vi "AE Save-Kamronn-Medtech.vi"(0 "error in (no error)":errorcluster, 2 "LstBox Refnum":refnum<vi>, 3 "Variant In":variant, 4 "Action":T1=enum."Save Listbox") -> (7 "error out":errorcluster, 10 "Anything":variant)   [LabVIEW 2013, in "main.lvlib"]
uses:
  main.lvlib
  Controls/Enum Save Action Events.ctl
  Controls/SaveDataCluster.ctl
  Controls/Enum Variables.ctl
  <userlib>/_OpenG.lib/file/file.llb/Valid Path - Traditional__ogtk.vi
  <userlib>/_OpenG.lib/file/file.llb/File Exists - Scalar__ogtk.vi
  Globals/DataPathGlobalVariable.vi
  Globals/DataAcqRecordPathGlobal.vi
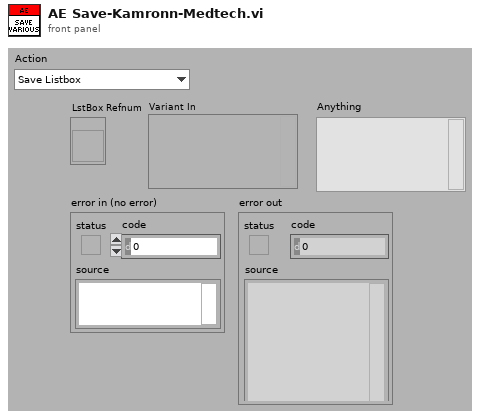
[diagram p1: front panel]
types:
  T1 = typedef "main.lvlib/Enum Save Action Events.ctl" = enum16{"LoadReportPath", "SaveReportPath", "Load Graph Path", "Save Graph Path", "LoadDataPath", "SaveDataPath", "Load Template Path", "Save Template Path", "Load PressureFactor", "Save PressureFactor", "Init", "Load Listbox", "Save Listbox", "LoadHospInfo", "SaveHospInfo", "Load DICOM Activation", "Save DICOM Activation", "LoadDICOMInfoWL", "SaveDICOMInfoWL", "LoadDICOMInfoPACS", "SaveDICOMInfoPACS", "Load ArmCalcMethod", "Save ArmCalcMethod", "LoadItemTags", "SaveItemTags", "LoadDICOMEncoding", "SaveDICOMEncoding", "LoadJournalType", "SaveJournalType", "LoadAcqFilterType", "SaveAcqFilterType", "Load Sequence", "Save Sequence", "Load Acquisition Mode", "Save Acquisition Mode", "Load General Settings", "Save General Settings", "Load Language", "Save Language", "Load Dicom Tags", "Save Dicom Tags", "Load BT Serial", "Save BT Serial", "Load BT License", "Save BT License"}
  T2 = typedef "main.lvlib/SaveDataCluster.ctl" = cluster{"HospInfo":cluster{"Name":string, "Address":string, "Department":string}, "Pressure":cluster{"Pressure":dbl}, "DataPath":cluster{"DataPath":path}, "ReportPath":cluster{"Path":path, "Name":string}, "DICOM Info WL":cluster{"port":i32, "AEtitle":string, "host":string, "remoteAE":string}, "DICOM Info PACS":cluster{"port":i32, "AEtitle":string, "host":string, "remoteAE":string}, "ArmCalcMethod":dbl, "itemTags":string[], "DicomEncoding":u16, "JournalType":u16, "General Settings":cluster{"Hyphenation":bool, "Language":u16, "CellStr1":string, "CellStr2":string}, "Dicom Tags":string[][], "BT Serial":cluster{"Serial Number":string, "Side":string, "Ignore?":bool}[], "BT License":cluster{"License":string, "Accepted Serials":string[]}}
  T3 = typedef "main.lvlib/Enum Variables.ctl" = enum16{"SetAcqFilter", "GetAcqFilter", "Set Filter", "Get Filter", "Set Height", "Get Height", "Set Recorded Height", "Get Recorded Height", "Set Blue Pressure", "Get Blue Pressure", "Set Red Pressure", "Get Red Pressure", "Init", "Reset Pressure", "Set Red Cursors", "Get Red Cursors", "Set Blue Cursors", "Get Blue Cursors", "Set Language", "Get Language", "Set Active Graphs", "Get ActiveGraphs", "Set Method", "Get Method", "Set Encryption", "Get Encryption", "Set ExcelVersion", "Get ExcelVersion", "Set DICOM Avail", "Get DICOM Avail", "Set DICOM Encode", "Get DICOM Encode", "Set JournalExport", "Get JournalExport", "Set Sequence", "Get Sequence", "Set DAQ Connected", "Get DAQ Connected", "Set Current Graph", "Get Current Graph", "Set General Settings", "Get Hyphenation", "Set Arm Calc Method", "Get Arm Calc Method", "Set Dicom Tags", "Get Dicom Tags", "Set BT Serial", "Get BT Serial", "Set BT Accepted Serials", "Get BT Accepted Serials", "Get BT License", "Set BT License"}
  T4 = cluster{"Name":string, "Address":string, "Department":string}
  T5 = cluster{"port":i32, "AEtitle":string, "host":string, "remoteAE":string}
  T6 = cluster{"Hyphenation":bool, "Language":u16, "CellStr1":string, "CellStr2":string}
  T7 = cluster{"Serial Number":string, "Side":string, "Ignore?":bool}[]
  T8 = cluster{"License":string, "Accepted Serials":string[]}
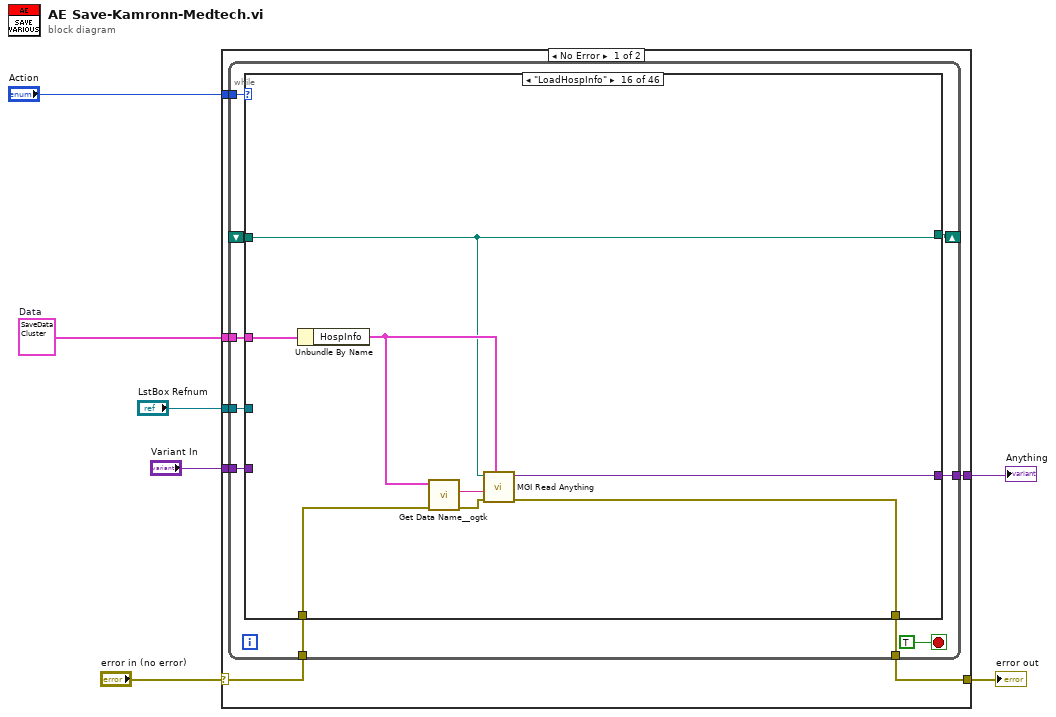
[diagram p0: block diagram]
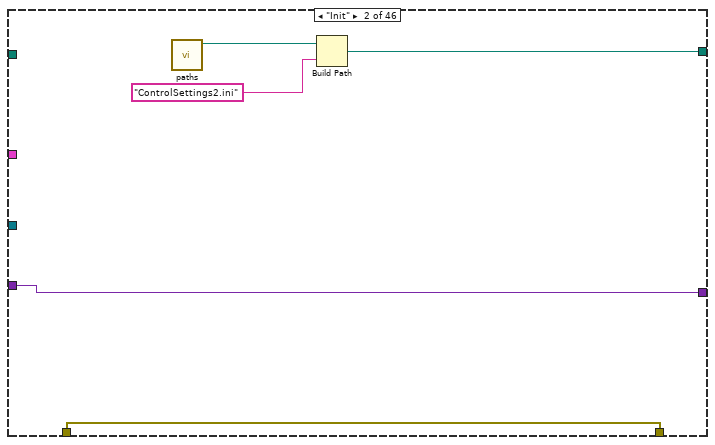
[diagram p3: hidden frame]
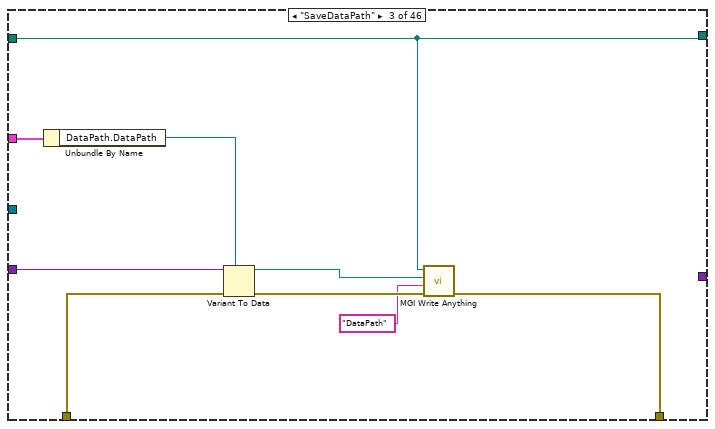
[diagram p4: hidden frame]
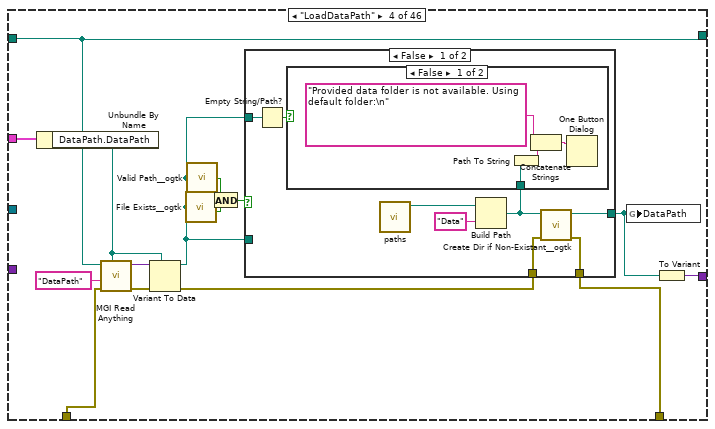
[diagram p5: hidden frame]
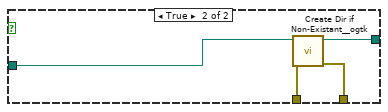
[diagram p7: hidden frame]
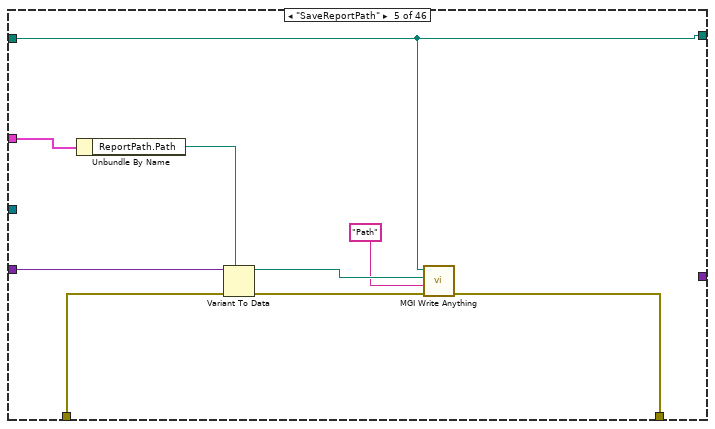
[diagram p8: hidden frame]
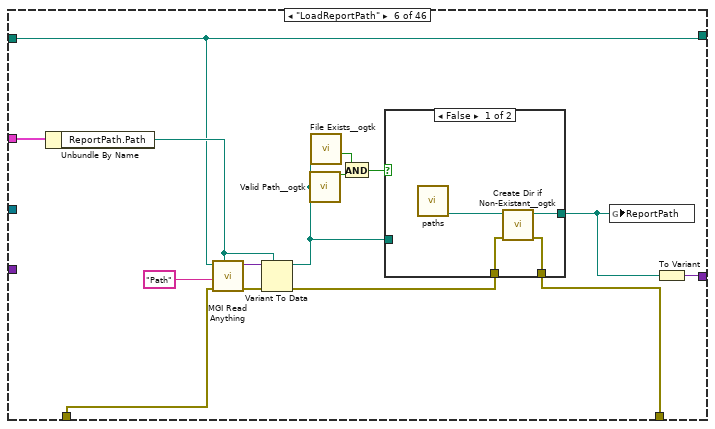
[diagram p9: hidden frame]
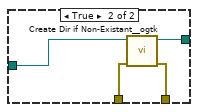
[diagram p10: hidden frame]
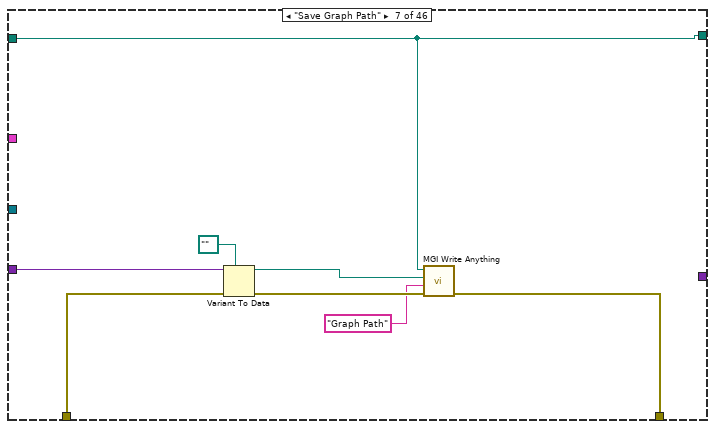
[diagram p11: hidden frame]
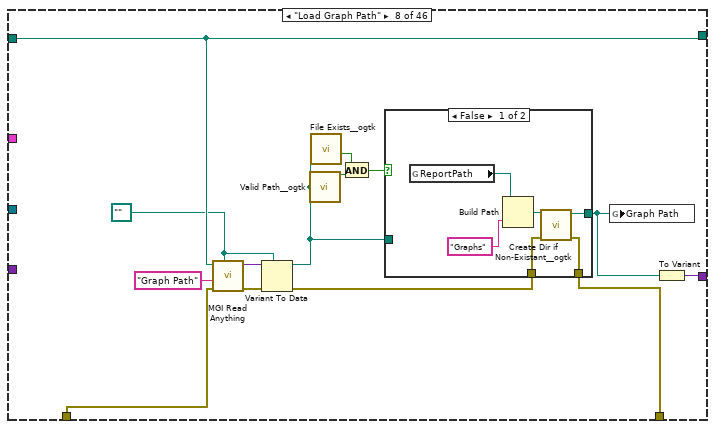
[diagram p12: hidden frame]
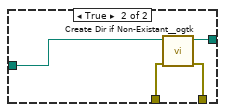
[diagram p13: hidden frame]
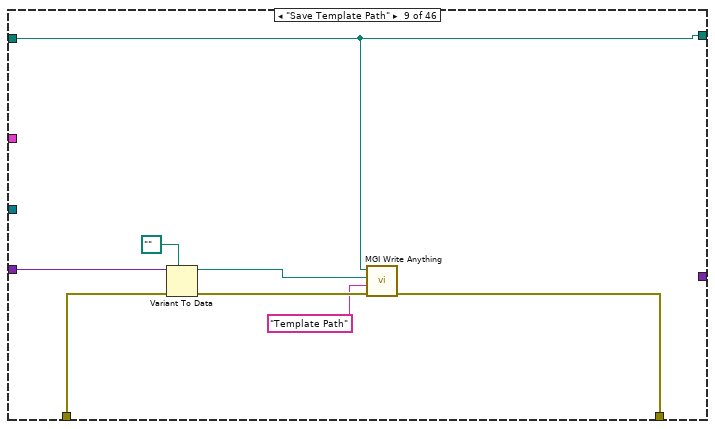
[diagram p14: hidden frame]
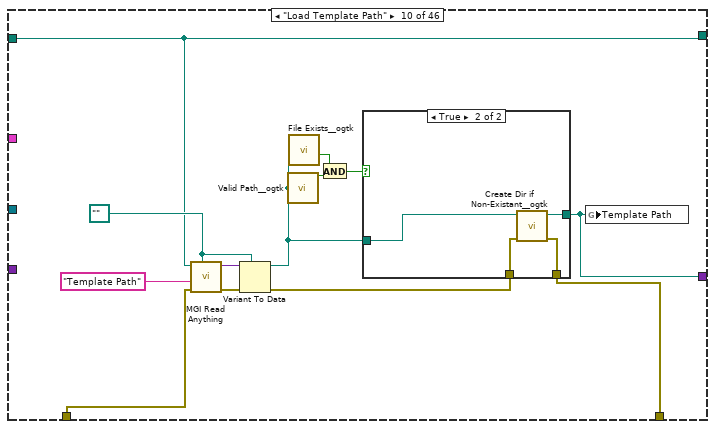
[diagram p15: hidden frame]
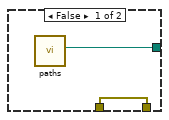
[diagram p16: hidden frame]
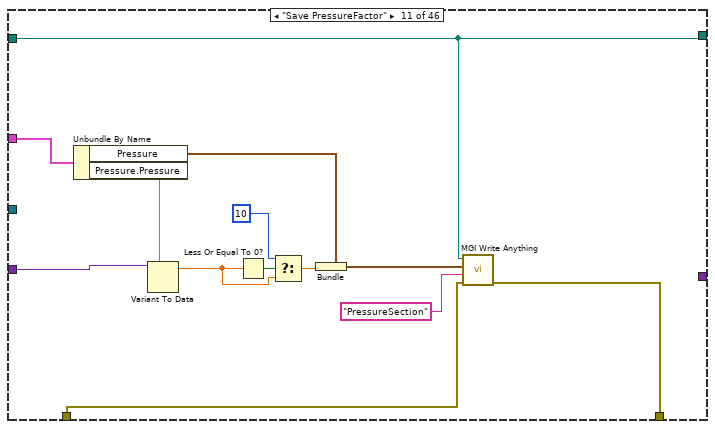
[diagram p17: hidden frame]
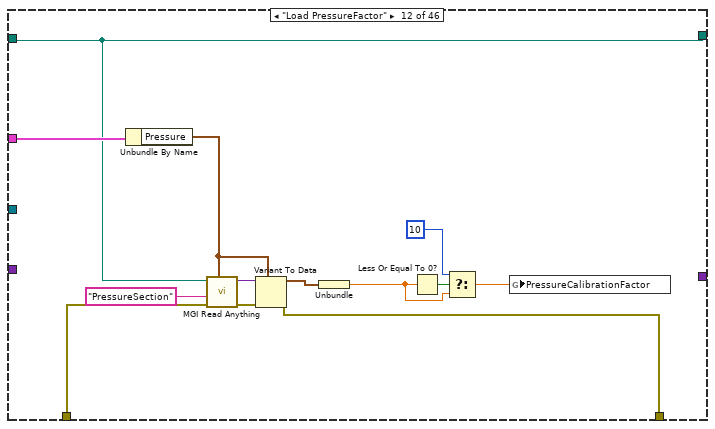
[diagram p18: hidden frame]
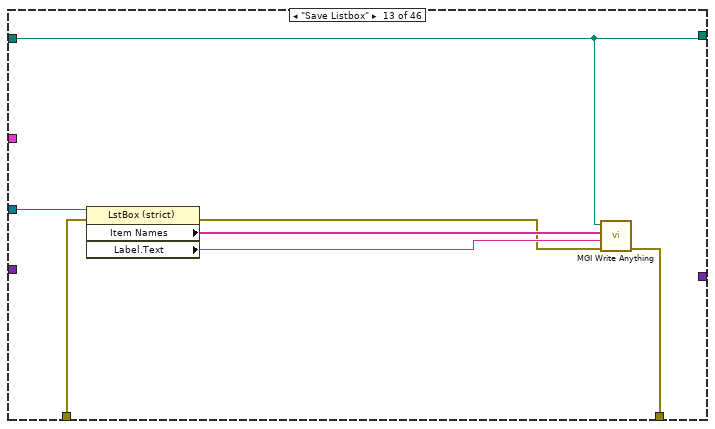
[diagram p19: hidden frame]
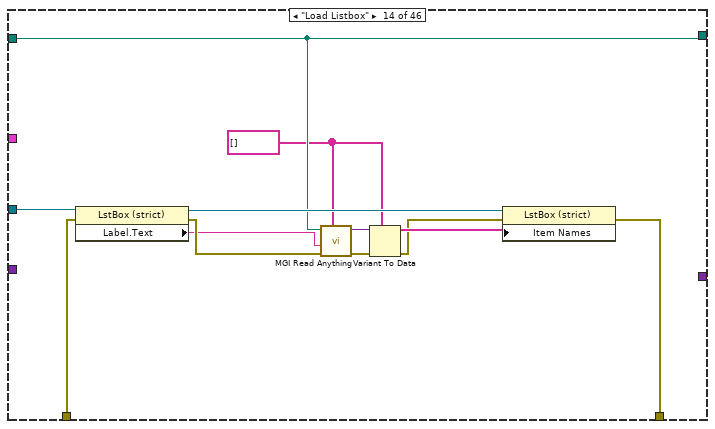
[diagram p20: hidden frame]
diagram:
  w2 = T2 {"HospInfo"={"Name"="", "Address"="", "Department"=""}, "Pressure"={"Pressure"=0.0}, "DataPath"={"DataPath"=path ""}, "ReportPath"={"Path"=path "", "Name"=""}, "DICOM Info WL"={"port"=0, "AEtitle"="", "host"="", "remoteAE"=""}, "DICOM Info PACS"={"port"=0, "AEtitle"="", "host"="", "remoteAE"=""}, "ArmCalcMethod"=0.0, "itemTags"=[], "DicomEncoding"=0, "JournalType"=0, "General Settings"={"Hyphenation"=FALSE, "Language"=0, "CellStr1"="", "CellStr2"=""}, "Dicom Tags"=[], "BT Serial"=[], "BT License"={"License"="", "Accepted Serials"=[]}}  # Data
  n1 = case shown="No Error" "error in (no error)" {
    selector: "error in (no error)" -> [w12 w535]
    tunnel: "Action" -> [w14 _]
    tunnel: "LstBox Refnum" -> [w13 _]
    tunnel: [w11 w535] -> w5
    tunnel: w2 -> [w10 _]
    tunnel: "Variant In" -> [w9 w534]
    tunnel: [w8 w534] -> w3
    frame No Error {
      n2 = while {
        tunnel: w14 -> [w23]
        tunnel: w13 -> [w22]
        tunnel: w12 -> [w21]
        tunnel: [w20] -> w11
        tunnel: w10 -> [w19]
        tunnel: w9 -> [w18]
        tunnel: [w17] -> w8
        shift-right: [w16] -> _
        shift-left: _ -> [w15]
        stop <- TRUE stop-if-true
        n3 = case shown="\"LoadHospInfo\"" w23 {
          tunnel: w22 -> [_ _ _ _ _ _ _ _ _ _ _ _ w196 w208 _ _ _ _ _ _ _ _ _ _ _ _ _ _ _ _ _ _ _ _ _ _ _ _ _ _ _ _ _ _ _ _]
          tunnel: w15 -> [w25 _ w33 w43 w74 w83 w107 w115 w137 w146 w164 w178 w192 w203 w209 w218 w230 w236 w241 w250 w256 w266 w276 w289 w294 w307 w330 w339 w345 w354 w359 w371 w373 w384 w395 w405 w418 w449 w457 w466 w480 w482 w500 w502 w518 w527]
          tunnel: w21 -> [w27 w32 w38 w51 w78 w92 w111 w124 w139 w149 w174 w184 w191 w202 w211 w222 w227 w237 w243 w249 w258 w265 w279 w288 w297 w308 w329 w340 w344 w355 w358 w372 w378 w387 w394 w404 w417 w448 w456 w465 w479 w485 w499 w505 w520 w529]
          tunnel: [w27 w32 w34 w49 w75 w90 w108 w122 w138 w148 w175 w183 w193 w199 w215 w219 w226 w235 w246 w251 w262 w267 w272 w284 w293 w309 w328 w336 w343 w351 w357 w365 w375 w385 w393 w402 w414 w444 w455 w463 w476 w483 w496 w503 w519 w528] -> w20
          tunnel: w19 -> [_ _ w40 w54 w80 w94 _ _ _ _ w171 w182 _ _ w217 w225 _ _ w247 w254 w263 w270 w281 w290 w299 w310 w327 w338 w342 w353 _ _ _ _ _ _ w416 w447 w454 _ w478 w487 w498 w507 w516 w526]
          tunnel: w18 -> [w26 w31 w41 _ w81 _ w112 _ w140 _ w169 _ _ _ w213 _ w231 _ w244 _ w260 _ w275 _ w292 _ w332 _ w347 _ w361 _ w381 _ w397 _ _ w450 w458 _ _ w488 _ w508 _ w530]
          tunnel: [w26 w31 _ w48 _ w89 _ w121 _ w147 _ _ _ _ w213 w220 _ w234 w244 w252 w260 w268 w275 w283 w292 w302 _ w337 _ w352 _ w364 _ _ _ w403 w407 _ _ w464 _ _ _ _ w513 _] -> w17
          tunnel: [w25 w30 w33 w43 w74 w83 w107 w115 w137 w146 w164 w178 w192 w203 w209 w218 w230 w236 w241 w250 w256 w266 w276 w289 w294 w307 w330 w339 w345 w354 w359 w371 w373 w384 w395 w405 w418 w449 w457 w466 w480 w482 w500 w502 w518 w527] -> w16
          frame Default {
          }
          frame "Init" {
            n4 = call "paths.vi"() -> ("PubAppData"=w29:path)  [unwired: 8 in, 3 out]
            n5 = Build Path(base path=w29, name or relative path="ControlSettings2.ini") -> (appended path=w30:path)
          }
          frame "SaveDataPath" {
            n6 = Unbundle By Name(w40) -> ("DataPath.DataPath"=w39:path)
            n7 = Variant To Data(error in=w38, type=w39, Variant=w41) -> (data=w35:path, error out=w37:errorcluster)
            n8 = call <userlib>:"MGI Write Anything.vi"("Error In"=w37, "Section Name (Name of \"Anything\")"="DataPath" ("Section Name (Name of \"Anything\")"), "Anything"=w35, "Path (dialog)"=w33) -> ("Error Out"=w34:errorcluster)  [unwired: 5 in, 2 out]
          }
          frame "LoadDataPath" {
            n9 = Unbundle By Name(w54) -> ("DataPath.DataPath"=w53:path)
            n10 = call <userlib>:"MGI Read Anything.vi"("Type of Anything"=w53, "Error In"=w51, "Section Name (Name of \"Type of Anything\")"="DataPath" ("Section Name (Name of \"Type of Anything\")"), "Path (dialog)"=w43) -> ("Error Out"=w56:errorcluster, "Anything"=w55:variant)  [unwired: 4 in, 2 out]
            n11 = Variant To Data(error in=w56, type=w53, Variant=w55) -> (data=w42:path, error out=w50:errorcluster)
            n12 = call-poly <userlib>:"File Exists__ogtk.vi"("file path"=w42) -> ("exists"=w45:bool)  [unwired: 6 in, 1 out]
            n13 = call-poly <userlib>:"Valid Path__ogtk.vi"("path"=w42) -> ("valid"=w44:bool)
            n14 = And(x=w44, y=w45) -> (x .and. y?=w46:bool)
            n15 = case shown="False" w46 {
              tunnel: w42 -> [_ w69]
              tunnel: [w63 w72] -> w47
              tunnel: w50 -> [w62 w71]
              tunnel: [w61 w70] -> w49
              tunnel: w42 -> [w59 _]
              frame False {
                n16 = Empty String/Path?(string/path=w59) -> (empty?=w58:bool)
                n17 = call "paths.vi"() -> ("PubAppData"=w60:path)  [unwired: 8 in, 3 out]
                n18 = Build Path(base path=w60, name or relative path="Data") -> (appended path=w57:path)
                n19 = case shown="False" w58 {
                  tunnel: w57 -> [w66 _]
                  frame False {
                    n20 = Path To String(path=w66) -> (string=w67:string)
                    n21 = Concatenate Strings("Provided data folder is not available. Using default folder:\n" ("message"), w67) -> (w65:string)
                    n22 = One Button Dialog(message=w65) -> ()  [unwired: 1 in, 1 out]
                  }
                  frame True {
                  }
                }
                n23 = call <userlib>:"Create Dir if Non-Existant__ogtk.vi"("error in (no error)"=w62, "Directory Path"=w57) -> ("error out"=w61:errorcluster, "dup Directory Path"=w63:path)  [unwired: 7 in, 1 out]
              }
              frame True {
                n24 = call <userlib>:"Create Dir if Non-Existant__ogtk.vi"("error in (no error)"=w71, "Directory Path"=w69) -> ("error out"=w70:errorcluster, "dup Directory Path"=w72:path)  [unwired: 7 in, 1 out]
              }
            }
            n25 = global write "DataPathGlobalVariable.vi" "DataPath"(w47) -> ()
            n26 = To Variant(anything=w47) -> (Variant=w48:variant)
          }
          frame "SaveReportPath" {
            n27 = Unbundle By Name(w80) -> ("ReportPath.Path"=w79:path)
            n28 = Variant To Data(error in=w78, type=w79, Variant=w81) -> (data=w76:path, error out=w77:errorcluster)
            n29 = call <userlib>:"MGI Write Anything.vi"("Error In"=w77, "Section Name (Name of \"Anything\")"="Path", "Anything"=w76, "Path (dialog)"=w74) -> ("Error Out"=w75:errorcluster)  [unwired: 5 in, 2 out]
          }
          frame "LoadReportPath" {
            n30 = Unbundle By Name(w94) -> ("ReportPath.Path"=w93:path)
            n31 = call <userlib>:"MGI Read Anything.vi"("Type of Anything"=w93, "Error In"=w92, "Section Name (Name of \"Type of Anything\")"="Path", "Path (dialog)"=w83) -> ("Error Out"=w96:errorcluster, "Anything"=w95:variant)  [unwired: 4 in, 2 out]
            n32 = Variant To Data(error in=w96, type=w93, Variant=w95) -> (data=w87:path, error out=w91:errorcluster)
            n33 = call-poly <userlib>:"Valid Path__ogtk.vi"("path"=w87) -> ("valid"=w84:bool)
            n34 = call-poly <userlib>:"File Exists__ogtk.vi"("file path"=w87) -> ("exists"=w85:bool)  [unwired: 6 in, 1 out]
            n35 = And(x=w85, y=w84) -> (x .and. y?=w86:bool)
            n36 = case shown="False" w86 {
              tunnel: w87 -> [_ w103]
              tunnel: [w100 w104] -> w88
              tunnel: w91 -> [w99 w102]
              tunnel: [w98 w101] -> w90
              frame False {
                n37 = call "paths.vi"() -> ("Journal Folder"=w97:path)  [unwired: 8 in, 3 out]
                n38 = call <userlib>:"Create Dir if Non-Existant__ogtk.vi"("error in (no error)"=w99, "Directory Path"=w97) -> ("error out"=w98:errorcluster, "dup Directory Path"=w100:path)  [unwired: 7 in, 1 out]
              }
              frame True {
                n39 = call <userlib>:"Create Dir if Non-Existant__ogtk.vi"("error in (no error)"=w102, "Directory Path"=w103) -> ("error out"=w101:errorcluster, "dup Directory Path"=w104:path)  [unwired: 7 in, 1 out]
              }
            }
            n40 = global write "DataPathGlobalVariable.vi" "ReportPath"(w88) -> ()
            n41 = To Variant(anything=w88) -> (Variant=w89:variant)
          }
          frame "Save Graph Path" {
            n42 = Variant To Data(error in=w111, type=path "", Variant=w112) -> (data=w109:path, error out=w110:errorcluster)
            n43 = call <userlib>:"MGI Write Anything.vi"("Error In"=w110, "Section Name (Name of \"Anything\")"="Graph Path", "Anything"=w109, "Path (dialog)"=w107) -> ("Error Out"=w108:errorcluster)  [unwired: 5 in, 2 out]
          }
          frame "Load Graph Path" {
            w113 = path ""
            n44 = call <userlib>:"MGI Read Anything.vi"("Type of Anything"=w113, "Error In"=w124, "Section Name (Name of \"Type of Anything\")"="Graph Path", "Path (dialog)"=w115) -> ("Error Out"=w126:errorcluster, "Anything"=w125:variant)  [unwired: 4 in, 2 out]
            n45 = Variant To Data(error in=w126, type=w113, Variant=w125) -> (data=w119:path, error out=w123:errorcluster)
            n46 = call-poly <userlib>:"Valid Path__ogtk.vi"("path"=w119) -> ("valid"=w116:bool)
            n47 = call-poly <userlib>:"File Exists__ogtk.vi"("file path"=w119) -> ("exists"=w117:bool)  [unwired: 6 in, 1 out]
            n48 = And(x=w117, y=w116) -> (x .and. y?=w118:bool)
            n49 = case shown="False" w118 {
              tunnel: w119 -> [_ w135]
              tunnel: [w132 w136] -> w120
              tunnel: w123 -> [w131 w134]
              tunnel: [w130 w133] -> w122
              frame False {
                n50 = global read "DataPathGlobalVariable.vi" "ReportPath"() -> (w127:path)
                n51 = Build Path(base path=w127, name or relative path="Graphs") -> (appended path=w129:path)
                n52 = call <userlib>:"Create Dir if Non-Existant__ogtk.vi"("error in (no error)"=w131, "Directory Path"=w129) -> ("error out"=w130:errorcluster, "dup Directory Path"=w132:path)  [unwired: 7 in, 1 out]
              }
              frame True {
                n53 = call <userlib>:"Create Dir if Non-Existant__ogtk.vi"("error in (no error)"=w134, "Directory Path"=w135) -> ("error out"=w133:errorcluster, "dup Directory Path"=w136:path)  [unwired: 7 in, 1 out]
              }
            }
            n54 = global write "DataPathGlobalVariable.vi" "Graph Path"(w120) -> ()
            n55 = To Variant(anything=w120) -> (Variant=w121:variant)
          }
          frame "Save Template Path" {
            n56 = Variant To Data(error in=w139, type=path "", Variant=w140) -> (data=w143:path, error out=w144:errorcluster)
            n57 = call <userlib>:"MGI Write Anything.vi"("Error In"=w144, "Section Name (Name of \"Anything\")"="Template Path", "Anything"=w143, "Path (dialog)"=w137) -> ("Error Out"=w138:errorcluster)  [unwired: 5 in, 2 out]
          }
          frame "Load Template Path" {
            w150 = path ""
            n58 = call <userlib>:"MGI Read Anything.vi"("Type of Anything"=w150, "Error In"=w149, "Section Name (Name of \"Type of Anything\")"="Template Path", "Path (dialog)"=w146) -> ("Error Out"=w157:errorcluster, "Anything"=w156:variant)  [unwired: 4 in, 2 out]
            n59 = Variant To Data(error in=w157, type=w150, Variant=w156) -> (data=w154:path, error out=w155:errorcluster)
            n60 = call-poly <userlib>:"Valid Path__ogtk.vi"("path"=w154) -> ("valid"=w151:bool)
            n61 = call-poly <userlib>:"File Exists__ogtk.vi"("file path"=w154) -> ("exists"=w152:bool)  [unwired: 6 in, 1 out]
            n62 = And(x=w152, y=w151) -> (x .and. y?=w153:bool)
            n63 = case shown="True" w153 {
              tunnel: w154 -> [_ w162]
              tunnel: [w159 w163] -> w147
              tunnel: w155 -> [w158 w161]
              tunnel: [w158 w160] -> w148
              frame False {
                n64 = call "paths.vi"() -> ("Journal Templates"=w159:path)  [unwired: 8 in, 3 out]
              }
              frame True {
                n65 = call <userlib>:"Create Dir if Non-Existant__ogtk.vi"("error in (no error)"=w161, "Directory Path"=w162) -> ("error out"=w160:errorcluster, "dup Directory Path"=w163:path)  [unwired: 7 in, 1 out]
              }
            }
            n66 = global write "DataPathGlobalVariable.vi" "Template Path"(w147) -> ()
          }
          frame "Save PressureFactor" {
            n67 = Unbundle By Name(w171) -> ("Pressure"=w168:cluster{"Pressure":dbl}, "Pressure.Pressure"=w170:dbl)
            n68 = Variant To Data(type=w170, Variant=w169) -> (data=w165:dbl)  [unwired: 1 in, 1 out]
            n69 = Less Or Equal To 0?(x=w165) -> (x <= 0?=w166:bool)
            n70 = Select(t=10, s=w166, f=w165) -> (s? t:f=w167:dbl)
            n71 = Bundle(cluster=w168, "Pressure"=w167) -> (w173:cluster{"Pressure":dbl})
            n72 = call <userlib>:"MGI Write Anything.vi"("Error In"=w174, "Section Name (Name of \"Anything\")"="PressureSection" ("Section Name (Name of \"Anything\")"), "Anything"=w173, "Path (dialog)"=w164) -> ("Error Out"=w175:errorcluster)  [unwired: 5 in, 2 out]
          }
          frame "Load PressureFactor" {
            n73 = Unbundle By Name(w182) -> ("Pressure"=w181:cluster{"Pressure":dbl})
            n74 = call <userlib>:"MGI Read Anything.vi"("Type of Anything"=w181, "Error In"=w184, "Section Name (Name of \"Type of Anything\")"="PressureSection" ("Section Name (Name of \"Anything\")"), "Path (dialog)"=w178) -> ("Error Out"=w189:errorcluster, "Anything"=w188:variant)  [unwired: 4 in, 2 out]
            n75 = Variant To Data(error in=w189, type=w181, Variant=w188) -> (data=w180:cluster{"Pressure":dbl}, error out=w183:errorcluster)
            n76 = Unbundle(w180) -> ("Pressure"=w179:dbl)
            n77 = Less Or Equal To 0?(x=w179) -> (x <= 0?=w187:bool)
            n78 = Select(t=10, s=w187, f=w179) -> (s? t:f=w185:dbl)
            n79 = global write "DataAcqRecordPathGlobal.vi" "PressureCalibrationFactor"(w185) -> ()
          }
          frame "Save Listbox" {
            n80 = property class="LstBox (strict)"(reference=w196, error in=w191) -> (error out=w190:errorcluster, "Item Names"=w194:string[], "Label.Text"=w195:string)  [unwired: 1 out]
            n81 = call <userlib>:"MGI Write Anything.vi"("Error In"=w190, "Section Name (Name of \"Anything\")"=w195, "Anything"=w194, "Path (dialog)"=w192) -> ("Error Out"=w193:errorcluster)  [unwired: 5 in, 2 out]
          }
          frame "Load Listbox" {
            w198 = string[] [] ("Item Names")
            n82 = property class="LstBox (strict)"(reference=w208, error in=w202) -> (reference out=w205:refnum<vi>, error out=w201:errorcluster, "Label.Text"=w197:string)
            n83 = call <userlib>:"MGI Read Anything.vi"("Type of Anything"=w198, "Error In"=w201, "Section Name (Name of \"Type of Anything\")"=w197, "Path (dialog)"=w203) -> ("Error Out"=w207:errorcluster, "Anything"=w206:variant)  [unwired: 4 in, 2 out]
            n84 = Variant To Data(error in=w207, type=w198, Variant=w206) -> (data=w204:string[], error out=w200:errorcluster)
            n85 = property class="LstBox (strict)"(reference=w205, error in=w200, "Item Names"=w204) -> (error out=w199:errorcluster)  [unwired: 1 out]
          }
          frame "SaveHospInfo" {
            n86 = Unbundle By Name(w217) -> ("HospInfo"=w212:T4)
            n87 = Variant To Data(error in=w211, type=w212, Variant=w213) -> (data=w214:T4, error out=w210:errorcluster)
            n88 = call <userlib>:"Get Data Name__ogtk.vi"("Data"=w212) -> ("Data Name"=w216:string)  [unwired: 8 in, 2 out]
            n89 = call <userlib>:"MGI Write Anything.vi"("Error In"=w210, "Section Name (Name of \"Anything\")"=w216, "Anything"=w214, "Path (dialog)"=w209) -> ("Error Out"=w215:errorcluster)  [unwired: 5 in, 2 out]
          }
          frame "LoadHospInfo" {
            n90 = Unbundle By Name(w225) -> ("HospInfo"=w221:T4)
            n91 = call <userlib>:"Get Data Name__ogtk.vi"("error in (no error)"=w222, "Data"=w221) -> ("error out"=w223:errorcluster, "Data Name"=w224:string)  [unwired: 7 in, 1 out]
            n92 = call <userlib>:"MGI Read Anything.vi"("Type of Anything"=w221, "Error In"=w223, "Section Name (Name of \"Type of Anything\")"=w224, "Path (dialog)"=w218) -> ("Error Out"=w219:errorcluster, "Anything"=w220:variant)  [unwired: 4 in, 2 out]
          }
          frame "Save DICOM Activation" {
            n93 = call "Encrypt.vi"("Input"="DICOM") -> ("Output"=w228:string)  [unwired: 10 in]
            n94 = call <userlib>:"MGI Write Anything.vi"("Error In"=w227, "Section Name (Name of \"Anything\")"=w228, "Anything"=w231, "Path (dialog)"=w230) -> ("Error Out"=w226:errorcluster)  [unwired: 5 in, 2 out]
          }
          frame "Load DICOM Activation" {
            n95 = call "Encrypt.vi"("Input"="DICOM") -> ("Output"=w232:string)  [unwired: 10 in]
            n96 = call <userlib>:"MGI Read Anything.vi"("Type of Anything"="", "Error In"=w237, "Section Name (Name of \"Type of Anything\")"=w232, "Path (dialog)"=w236) -> ("Error Out"=w235:errorcluster, "Anything"=w234:variant)  [unwired: 4 in, 2 out]
          }
          frame "SaveDICOMInfoWL" {
            n97 = Unbundle By Name(w247) -> ("DICOM Info WL"=w240:T5)
            n98 = Variant To Data(error in=w243, type=w240, Variant=w244) -> (data=w245:T5, error out=w242:errorcluster)
            n99 = call <userlib>:"MGI Write Anything.vi"("Error In"=w242, "Section Name (Name of \"Anything\")"="DICOM Info WL", "Anything"=w245, "Path (dialog)"=w241) -> ("Error Out"=w246:errorcluster)  [unwired: 5 in, 2 out]
          }
          frame "LoadDICOMInfoWL" {
            n100 = Unbundle By Name(w254) -> ("DICOM Info WL"=w253:T5)
            n101 = call <userlib>:"MGI Read Anything.vi"("Type of Anything"=w253, "Error In"=w249, "Section Name (Name of \"Type of Anything\")"="DICOM Info WL", "Path (dialog)"=w250) -> ("Error Out"=w251:errorcluster, "Anything"=w252:variant)  [unwired: 4 in, 2 out]
          }
          frame "SaveDICOMInfoPACS" {
            n102 = Unbundle By Name(w263) -> ("DICOM Info PACS"=w259:T5)
            n103 = Variant To Data(error in=w258, type=w259, Variant=w260) -> (data=w261:T5, error out=w257:errorcluster)
            n104 = call <userlib>:"MGI Write Anything.vi"("Error In"=w257, "Section Name (Name of \"Anything\")"="DICOM Info PACS", "Anything"=w261, "Path (dialog)"=w256) -> ("Error Out"=w262:errorcluster)  [unwired: 5 in, 2 out]
          }
          frame "LoadDICOMInfoPACS" {
            n105 = Unbundle By Name(w270) -> ("DICOM Info PACS"=w269:T5)
            n106 = call <userlib>:"MGI Read Anything.vi"("Type of Anything"=w269, "Error In"=w265, "Section Name (Name of \"Type of Anything\")"="DICOM Info PACS", "Path (dialog)"=w266) -> ("Error Out"=w267:errorcluster, "Anything"=w268:variant)  [unwired: 4 in, 2 out]
          }
          frame "Save ArmCalcMethod" {
            n107 = Unbundle By Name(w281) -> ("ArmCalcMethod"=w280:dbl)
            n108 = Variant To Data(error in=w279, type=w280, Variant=w275) -> (data=w271:dbl, error out=w278:errorcluster)
            n109 = call <userlib>:"MGI Write Anything.vi"("Error In"=w278, "Section Name (Name of \"Anything\")"="ArmCalcMethod", "Anything"=w271, "Path (dialog)"=w276) -> ("Error Out"=w273:errorcluster)  [unwired: 5 in, 2 out]
            n110 = call "AE Variables.vi"("VariantIn"=w271, "error in (no error)"=w273, "Action"=Enum_Variables."Set Arm Calc Method") -> ("error out"=w272:errorcluster)  [unwired: 9 in, 7 out]
          }
          frame "Load ArmCalcMethod" {
            n111 = Unbundle By Name(w290) -> ("ArmCalcMethod"=w287:dbl)
            n112 = call <userlib>:"MGI Read Anything.vi"("Type of Anything"=w287, "Error In"=w288, "Section Name (Name of \"Type of Anything\")"="ArmCalcMethod", "Path (dialog)"=w289) -> ("Error Out"=w285:errorcluster, "Anything"=w283:variant)  [unwired: 4 in, 2 out]
            n113 = call "AE Variables.vi"("VariantIn"=w283, "error in (no error)"=w285, "Action"=Enum_Variables."Set Arm Calc Method") -> ("error out"=w284:errorcluster)  [unwired: 9 in, 7 out]
          }
          frame "SaveItemTags" {
            n114 = Unbundle By Name(w299) -> ("itemTags"=w298:string[])
            n115 = Variant To Data(error in=w297, type=w298, Variant=w292) -> (data=w291:string[], error out=w296:errorcluster)
            n116 = call <userlib>:"MGI Write Anything.vi"("Error In"=w296, "Section Name (Name of \"Anything\")"="itemTags", "Anything"=w291, "Path (dialog)"=w294) -> ("Error Out"=w293:errorcluster)  [unwired: 5 in, 2 out]
          }
          frame "LoadItemTags" {
            n117 = Unbundle By Name(w310) -> ("itemTags"=w306:string[])
            n118 = call <userlib>:"MGI Read Anything.vi"("Type of Anything"=w306, "Error In"=w308, "Section Name (Name of \"Type of Anything\")"="itemTags", "Path (dialog)"=w307) -> ("Error Out"=w309:errorcluster, "Anything"=w303:variant)  [unwired: 4 in, 2 out]
            n119 = Variant To Data(type=w306, Variant=w303) -> (data=w301:string[])  [unwired: 1 in, 1 out]
            n120 = Empty Array?(array=w301) -> (empty?=w305:bool)
            n121 = case shown="False" w305 {
              tunnel: string[] ["PatientsName", "PatientId", "AccessionNumber", "ReferringPhysiciansName", "RequestingPhysician", "OperatorsName", "RequestedProcedureDescription", "RequestedProcedureId", "StudyInstanceUid", "StudyId", "SeriesInstanceUid", "PatientsBirthDate"] -> [w314 w325]
              tunnel: [w312 w324] -> w302
              tunnel: w301 -> [w313 _]
              frame False {
                n122 = for {
                  tunnel: w314 -> [w316] mode=indexing
                  shift-right: [w317] -> w311
                  shift-left: w313 -> [w318]
                  n123 = Search 1D Array(1D array=w318, element=w316) -> (index of element=w319:i32)  [unwired: 1 in]
                  n124 = Less Than 0?(x=w319) -> (x < 0?=w315:bool)
                  n125 = case shown="True" w315 {
                    tunnel: w318 -> [w320 w323]
                    tunnel: [w320 w322] -> w317
                    tunnel: w316 -> [_ w321]
                    frame False {
                    }
                    frame True {
                      n126 = Build Array (concatenate)(w323, w321) -> (w322:string[])
                    }
                  }
                }
                n127 = To Variant(anything=w311) -> (Variant=w312:variant)
              }
              frame True {
                n128 = To Variant(anything=w325) -> (Variant=w324:variant)
              }
            }
          }
          frame "SaveDICOMEncoding" {
            n129 = Unbundle By Name(w327) -> ("DicomEncoding"=w326:u16)
            n130 = Variant To Data(type=w326, Variant=w332) -> (data=w333:u16)  [unwired: 1 in, 1 out]
            n131 = call <userlib>:"MGI Write Anything.vi"("Error In"=w329, "Section Name (Name of \"Anything\")"="DicomEncoding", "Anything"=w333, "Path (dialog)"=w330) -> ("Error Out"=w328:errorcluster)  [unwired: 5 in, 2 out]
          }
          frame "LoadDICOMEncoding" {
            n132 = Unbundle By Name(w338) -> ("DicomEncoding"=w335:u16)
            n133 = call <userlib>:"MGI Read Anything.vi"("Type of Anything"=w335, "Error In"=w340, "Section Name (Name of \"Type of Anything\")"="DicomEncoding", "Path (dialog)"=w339) -> ("Error Out"=w336:errorcluster, "Anything"=w337:variant)  [unwired: 4 in, 2 out]
          }
          frame "SaveJournalType" {
            n134 = Unbundle By Name(w342) -> ("JournalType"=w341:u16)
            n135 = Variant To Data(type=w341, Variant=w347) -> (data=w348:u16)  [unwired: 1 in, 1 out]
            n136 = call <userlib>:"MGI Write Anything.vi"("Error In"=w344, "Section Name (Name of \"Anything\")"="JournalExportType", "Anything"=w348, "Path (dialog)"=w345) -> ("Error Out"=w343:errorcluster)  [unwired: 5 in, 2 out]
          }
          frame "LoadJournalType" {
            n137 = Unbundle By Name(w353) -> ("JournalType"=w350:u16)
            n138 = call <userlib>:"MGI Read Anything.vi"("Type of Anything"=w350, "Error In"=w355, "Section Name (Name of \"Type of Anything\")"="JournalExportType", "Path (dialog)"=w354) -> ("Error Out"=w351:errorcluster, "Anything"=w352:variant)  [unwired: 4 in, 2 out]
          }
          frame "SaveAcqFilterType" {
            n139 = Variant To Data(type=0, Variant=w361) -> (data=w362:i32)  [unwired: 1 in, 1 out]
            n140 = call <userlib>:"MGI Write Anything.vi"("Error In"=w358, "Section Name (Name of \"Anything\")"="AcqFilterType", "Anything"=w362, "Path (dialog)"=w359) -> ("Error Out"=w357:errorcluster)  [unwired: 5 in, 2 out]
          }
          frame "LoadAcqFilterType" {
            w363 = 0
            n141 = call <userlib>:"MGI Read Anything.vi"("Type of Anything"=w363, "Error In"=w372, "Section Name (Name of \"Type of Anything\")"="AcqFilterType", "Path (dialog)"=w371) -> ("Error Out"=w368:errorcluster, "Anything"=w364:variant)  [unwired: 4 in, 2 out]
            n142 = Variant To Data(error in=w368, type=w363, Variant=w364) -> (data=w367:i32, error out=w366:errorcluster)
            n143 = call "AE Variables.vi"("VariantIn"=w367, "error in (no error)"=w366, "Action"=Enum_Variables."SetAcqFilter") -> ("error out"=w365:errorcluster)  [unwired: 9 in, 7 out]
          }
          frame "Save Sequence" {
            n144 = Variant To Data(error in=w378, type="", Variant=w381) -> (data=w374:string, error out=w379:errorcluster)
            n145 = call <userlib>:"MGI Write Anything.vi"("Error In"=w379, "Section Name (Name of \"Anything\")"="Sequence", "Anything"=w374, "Path (dialog)"=w373) -> ("Error Out"=w376:errorcluster)  [unwired: 5 in, 2 out]
            n146 = call "AE Variables.vi"("VariantIn"=w374, "error in (no error)"=w376, "Action"=Enum_Variables."Set Sequence") -> ("error out"=w375:errorcluster)  [unwired: 9 in, 7 out]
          }
          frame "Load Sequence" {
            w386 = ""
            n147 = call <userlib>:"MGI Read Anything.vi"("Type of Anything"=w386, "Error In"=w387, "Section Name (Name of \"Type of Anything\")"="Sequence", "Path (dialog)"=w384) -> ("Error Out"=w391:errorcluster, "Anything"=w388:variant)  [unwired: 4 in, 2 out]
            n148 = Variant To Data(error in=w391, type=w386, Variant=w388) -> (data=w390:string, error out=w389:errorcluster)
            n149 = call "AE Variables.vi"("VariantIn"=w390, "error in (no error)"=w389, "Action"=Enum_Variables."Set Sequence") -> ("error out"=w385:errorcluster)  [unwired: 9 in, 7 out]
          }
          frame "Save Acquisition Mode" {
            n150 = Variant To Data(error in=w394, type=TRUE, Variant=w397) -> (data=w398:bool, error out=w399:errorcluster)
            n151 = call <userlib>:"MGI Write Anything.vi"("Error In"=w399, "Section Name (Name of \"Anything\")"="Acquisition Mode", "Anything"=w398, "Path (dialog)"=w395) -> ("Error Out"=w393:errorcluster)  [unwired: 5 in, 2 out]
          }
          frame "Load Acquisition Mode" {
            n152 = call <userlib>:"MGI Read Anything.vi"("Type of Anything"=FALSE, "Error In"=w404, "Section Name (Name of \"Type of Anything\")"="Acquisition Mode", "Path (dialog)"=w405) -> ("Error Out"=w402:errorcluster, "Anything"=w403:variant)  [unwired: 4 in, 2 out]
          }
          frame "Load General Settings" {
            n153 = Unbundle By Name(w416) -> ("General Settings"=w415:T6)
            n154 = call <userlib>:"MGI Read Anything.vi"("Type of Anything"=w415, "Error In"=w417, "Section Name (Name of \"Type of Anything\")"="General Settings" ("Section Name (Name of \"Type of Anything\")"), "Path (dialog)"=w418) -> ("Error Out"=w411:errorcluster, "Found?"=w409:bool, "Anything"=w408:variant)  [unwired: 4 in, 1 out]
            n155 = case shown="False" w409 {
              tunnel: w411 -> [w419 w442]
              tunnel: [w421 w442] -> w410
              tunnel: w408 -> [w422 w443]
              tunnel: [w420 w443] -> w407
              frame False {
                n156 = call "GetCountry.vi"() -> ("data"=w423:string)  [unwired: 11 in]
                n157 = case shown="\"DK\", \"DNK\"" w423 {
                  tunnel: w422 -> [w429 w435 w441]
                  tunnel: w419 -> [w426 w432 w438]
                  tunnel: [w425 w431 w437] -> w421
                  tunnel: [w424 w430 w436] -> w420
                  frame "DK", "DNK" {
                    n158 = call <userlib>:"Set Cluster Element by Name__ogtk.vi"("error in (no error)"=w426, "Element Name (\"\": New Element Data Name)"="Language" ("Element Name (\"\": New Element Data Name)"), "New Element Value"=0, "Cluster"=w429) -> ("error out"=w425:errorcluster, "VCluster out"=w424:variant)  [unwired: 5 in, 1 out]
                  }
                  frame "US", Default {
                    n159 = call <userlib>:"Set Cluster Element by Name__ogtk.vi"("error in (no error)"=w432, "Element Name (\"\": New Element Data Name)"="Language" ("Element Name (\"\": New Element Data Name)"), "New Element Value"=1, "Cluster"=w435) -> ("error out"=w431:errorcluster, "VCluster out"=w430:variant)  [unwired: 5 in, 1 out]
                  }
                  frame "FR", "FRA" {
                    n160 = call <userlib>:"Set Cluster Element by Name__ogtk.vi"("error in (no error)"=w438, "Element Name (\"\": New Element Data Name)"="Language" ("Element Name (\"\": New Element Data Name)"), "New Element Value"=2, "Cluster"=w441) -> ("error out"=w437:errorcluster, "VCluster out"=w436:variant)  [unwired: 5 in, 1 out]
                  }
                }
              }
              frame True {
              }
            }
            n161 = call "AE Variables.vi"("VariantIn"=w407, "error in (no error)"=w410, "Action"=Enum_Variables."Set General Settings") -> ("error out"=w414:errorcluster)  [unwired: 9 in, 7 out]
          }
          frame "Save General Settings" {
            n162 = Unbundle By Name(w447) -> ("General Settings"=w446:T6)
            n163 = Variant To Data(error in=w448, type=w446, Variant=w450) -> (data=w445:T6, error out=w451:errorcluster)
            n164 = call <userlib>:"MGI Write Anything.vi"("Error In"=w451, "Section Name (Name of \"Anything\")"="General Settings", "Anything"=w445, "Path (dialog)"=w449) -> ("Error Out"=w444:errorcluster)  [unwired: 5 in, 2 out]
          }
          frame "Save Language" {
            n165 = Unbundle By Name(w454) -> ("General Settings"=w453:T6)
            n166 = Variant To Data(error in=w456, type=w453, Variant=w458) -> (data=w459:T6, error out=w460:errorcluster)
            n167 = call <userlib>:"MGI Write Anything.vi"("Error In"=w460, "Section Name (Name of \"Anything\")"="Language", "Anything"=w459, "Path (dialog)"=w457) -> ("Error Out"=w455:errorcluster)  [unwired: 5 in, 2 out]
          }
          frame "Load Language" {
            n168 = call <userlib>:"MGI Read Anything.vi"("Type of Anything"=FALSE, "Error In"=w465, "Section Name (Name of \"Type of Anything\")"="Language", "Path (dialog)"=w466) -> ("Error Out"=w463:errorcluster, "Anything"=w464:variant)  [unwired: 4 in, 2 out]
          }
          frame "Load Dicom Tags" {
            n169 = Unbundle By Name(w478) -> ("Dicom Tags"=w475:string[][])
            n170 = call <userlib>:"MGI Read Anything.vi"("Type of Anything"=w475, "Error In"=w479, "Section Name (Name of \"Type of Anything\")"="Dicom Tags", "Path (dialog)"=w480) -> ("Error Out"=w474:errorcluster, "Anything"=w470:variant)  [unwired: 4 in, 2 out]
            n171 = Variant To Data(error in=w474, type=w475, Variant=w470) -> (data=w473:string[][], error out=w468:errorcluster)
            n172 = Empty Array?(array=w473) -> (empty?=w471:bool)
            n173 = Select(t=string[][] [["0010", "0010", "PatientName"], ["0010", "0020", "PatientID"]], s=w471, f=w470) -> (s? t:f=w469:variant)
            n174 = call "AE Variables.vi"("VariantIn"=w469, "error in (no error)"=w468, "Action"=Enum_Variables."Set Dicom Tags") -> ("error out"=w476:errorcluster)  [unwired: 9 in, 7 out]
          }
          frame "Save Dicom Tags" {
            n175 = Unbundle By Name(w487) -> ("Dicom Tags"=w484:string[][])
            n176 = Variant To Data(error in=w485, type=w484, Variant=w488) -> (data=w489:string[][], error out=w490:errorcluster)
            n177 = call <userlib>:"MGI Write Anything.vi"("Error In"=w490, "Section Name (Name of \"Anything\")"="Dicom Tags", "Anything"=w489, "Path (dialog)"=w482) -> ("Error Out"=w483:errorcluster)  [unwired: 5 in, 2 out]
          }
          frame "Load BT Serial" {
            n178 = Unbundle By Name(w498) -> ("BT Serial"=w495:T7)
            n179 = call <userlib>:"MGI Read Anything.vi"("Type of Anything"=w495, "Error In"=w499, "Section Name (Name of \"Type of Anything\")"="BT Serial", "Path (dialog)"=w500) -> ("Error Out"=w494:errorcluster, "Anything"=w493:variant)  [unwired: 4 in, 2 out]
            n180 = Variant To Data(error in=w494, type=w495, Variant=w493) -> (data=w491:T7, error out=w492:errorcluster)
            n181 = call "AE Variables.vi"("VariantIn"=w491, "error in (no error)"=w492, "Action"=Enum_Variables."Set BT Serial") -> ("error out"=w496:errorcluster)  [unwired: 9 in, 7 out]
          }
          frame "Save BT Serial" {
            n182 = Unbundle By Name(w507) -> ("BT Serial"=w504:T7)
            n183 = Variant To Data(error in=w505, type=w504, Variant=w508) -> (data=w509:T7, error out=w510:errorcluster)
            n184 = call <userlib>:"MGI Write Anything.vi"("Error In"=w510, "Section Name (Name of \"Anything\")"="BT Serial", "Anything"=w509, "Path (dialog)"=w502) -> ("Error Out"=w503:errorcluster)  [unwired: 5 in, 2 out]
          }
          frame "Load BT License" {
            n185 = Unbundle By Name(w516) -> ("BT License"=w515:T8)
            n186 = call <userlib>:"MGI Read Anything.vi"("Type of Anything"=w515, "Error In"=w520, "Section Name (Name of \"Type of Anything\")"="BT License", "Path (dialog)"=w518) -> ("Error Out"=w522:errorcluster, "Anything"=w521:variant)  [unwired: 4 in, 2 out]
            n187 = Variant To Data(error in=w522, type=w515, Variant=w521) -> (data=w513:T8, error out=w511:errorcluster)
            n188 = Unbundle By Name(w513) -> ("License"=w514:string)
            n189 = Unbundle By Name(w513) -> ("Accepted Serials"=w512:string[])
            n190 = call "AE Variables.vi"("VariantIn"=w512, "error in (no error)"=w511, "Action"=Enum_Variables."Set BT Accepted Serials") -> ("error out"=w519:errorcluster)  [unwired: 9 in, 7 out]
            n191 = call "AE Variables.vi"("VariantIn"=w514, "Action"=Enum_Variables."Set BT License") -> ()  [unwired: 10 in, 8 out]
          }
          frame "Save BT License" {
            n192 = Unbundle By Name(w526) -> ("BT License"=w525:T8)
            n193 = Variant To Data(error in=w529, type=w525, Variant=w530) -> (data=w532:T8, error out=w533:errorcluster)
            n194 = call <userlib>:"MGI Write Anything.vi"("Error In"=w533, "Section Name (Name of \"Anything\")"="BT License", "Anything"=w532, "Path (dialog)"=w527) -> ("Error Out"=w528:errorcluster)  [unwired: 5 in, 2 out]
          }
        }
      }
    }
    frame Error {
    }
  }
  "error out" <- w5
  "Anything" <- w3
